vi "CARICA GRAFICI.vi"(0 "TRIFASE?":bool, 1 "N°curva":i32, 2 "TERMICA?":bool, 5 "indici":T2, 7 "CURVE SINGOLE IN":T3, 9 "dati":string[][](array[string]), 11 "filtra\nNPSH":bool, 12 "Cluster filtro":cluster{"index":i32, "length":i32}, 13 "Cluster":T1={"scelta grafico QH"=0, "scelta grafico QP"=1, "scelta grafico Qeta"=0, "scelta grafico temperature"=0} {"scelta grafico QH" items=["Q-Htot", "Q(n)-Htot(n)"]; "scelta grafico QP" items=["Q-P1", "Q-P2", "Q-P3", "Q(n)-P1(n)", "Q(n)-P2(n)", "Q(n)-P2(n Ps)", "Q(n)-P3(n)"]; "scelta grafico Qeta" items=["Q-EtaP", "Q-EtaGr", "Q(n)-Etap(n)", "Q(n)-EtaGr(n)"]; "scelta grafico temperature" items=["DT", "DTaux", "TC1", "TC2"]}, 14 "Grafico generico":cluster{"X":i32, "Y":i32}) -> (3 "Temperature":cluster{"X":dbl[], "Y":dbl[]}[](array[cluster]), 4 "Cluster graph":T4, 6 "curve idrauliche":cluster{"X":dbl[], "Y":dbl[]}[](array[cluster]), 8 "Collaudo da graficare":T3, 10 "rendimenti/Pot":cluster{"X":dbl[], "Y":dbl[]}[](array[cluster]), 15 "CURVE SINGOLE OUT":T3)   [LabVIEW 2019]
uses:
  TypeDef/Curve singole.ctl
  TypeDef/Indici.ctl
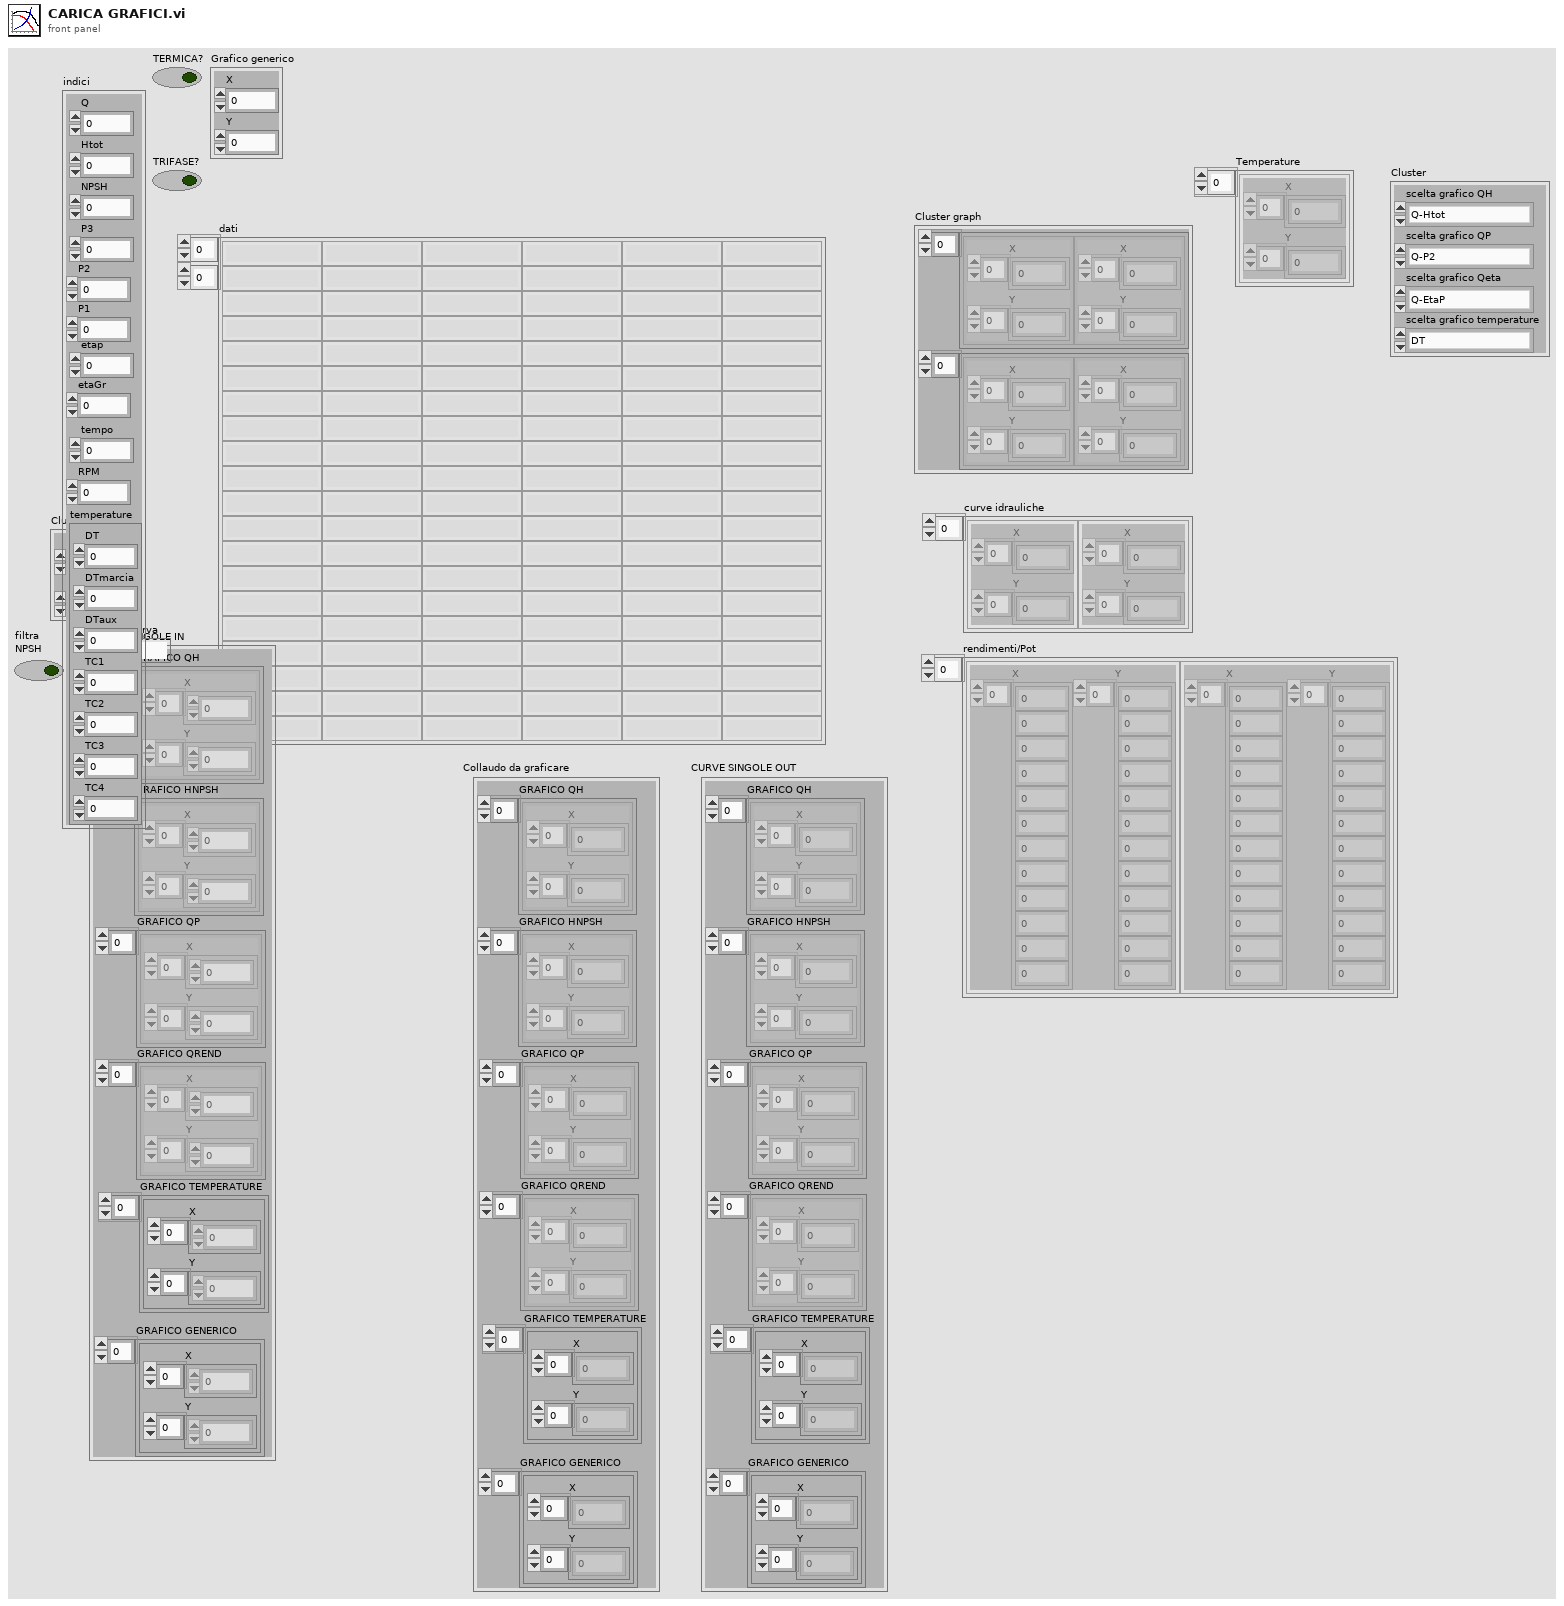
[diagram p1: front panel]
types:
  T1 = cluster{"scelta grafico QH":u16, "scelta grafico QP":u16, "scelta grafico Qeta":u16, "scelta grafico temperature":u16}
  T2 = typedef "Indici.ctl" = cluster{"Q":i32, "Htot":i32, "NPSH":i32, "P3":i32, "etap":i32, "temperature":cluster{"DT":i32, "DTmarcia":i32, "DTaux":i32, "TC1":i32, "TC2":i32, "TC3":i32, "TC4":i32}, "tempo":i32, "P2":i32, "P1":i32, "etaGr":i32, "RPM":i32}
  T3 = typedef "Curve singole.ctl" = cluster{"GRAFICO QH":cluster{"X":dbl[], "Y":dbl[]}[], "GRAFICO HNPSH":cluster{"X":dbl[], "Y":dbl[]}[], "GRAFICO QP":cluster{"X":dbl[], "Y":dbl[]}[], "GRAFICO QREND":cluster{"X":dbl[], "Y":dbl[]}[], "GRAFICO TEMPERATURE":cluster{"X":dbl[], "Y":dbl[]}[], "GRAFICO GENERICO":cluster{"X":dbl[], "Y":dbl[]}[]}
  T4 = cluster{cluster{"X":dbl[], "Y":dbl[]}[], cluster{"X":dbl[], "Y":dbl[]}[]}
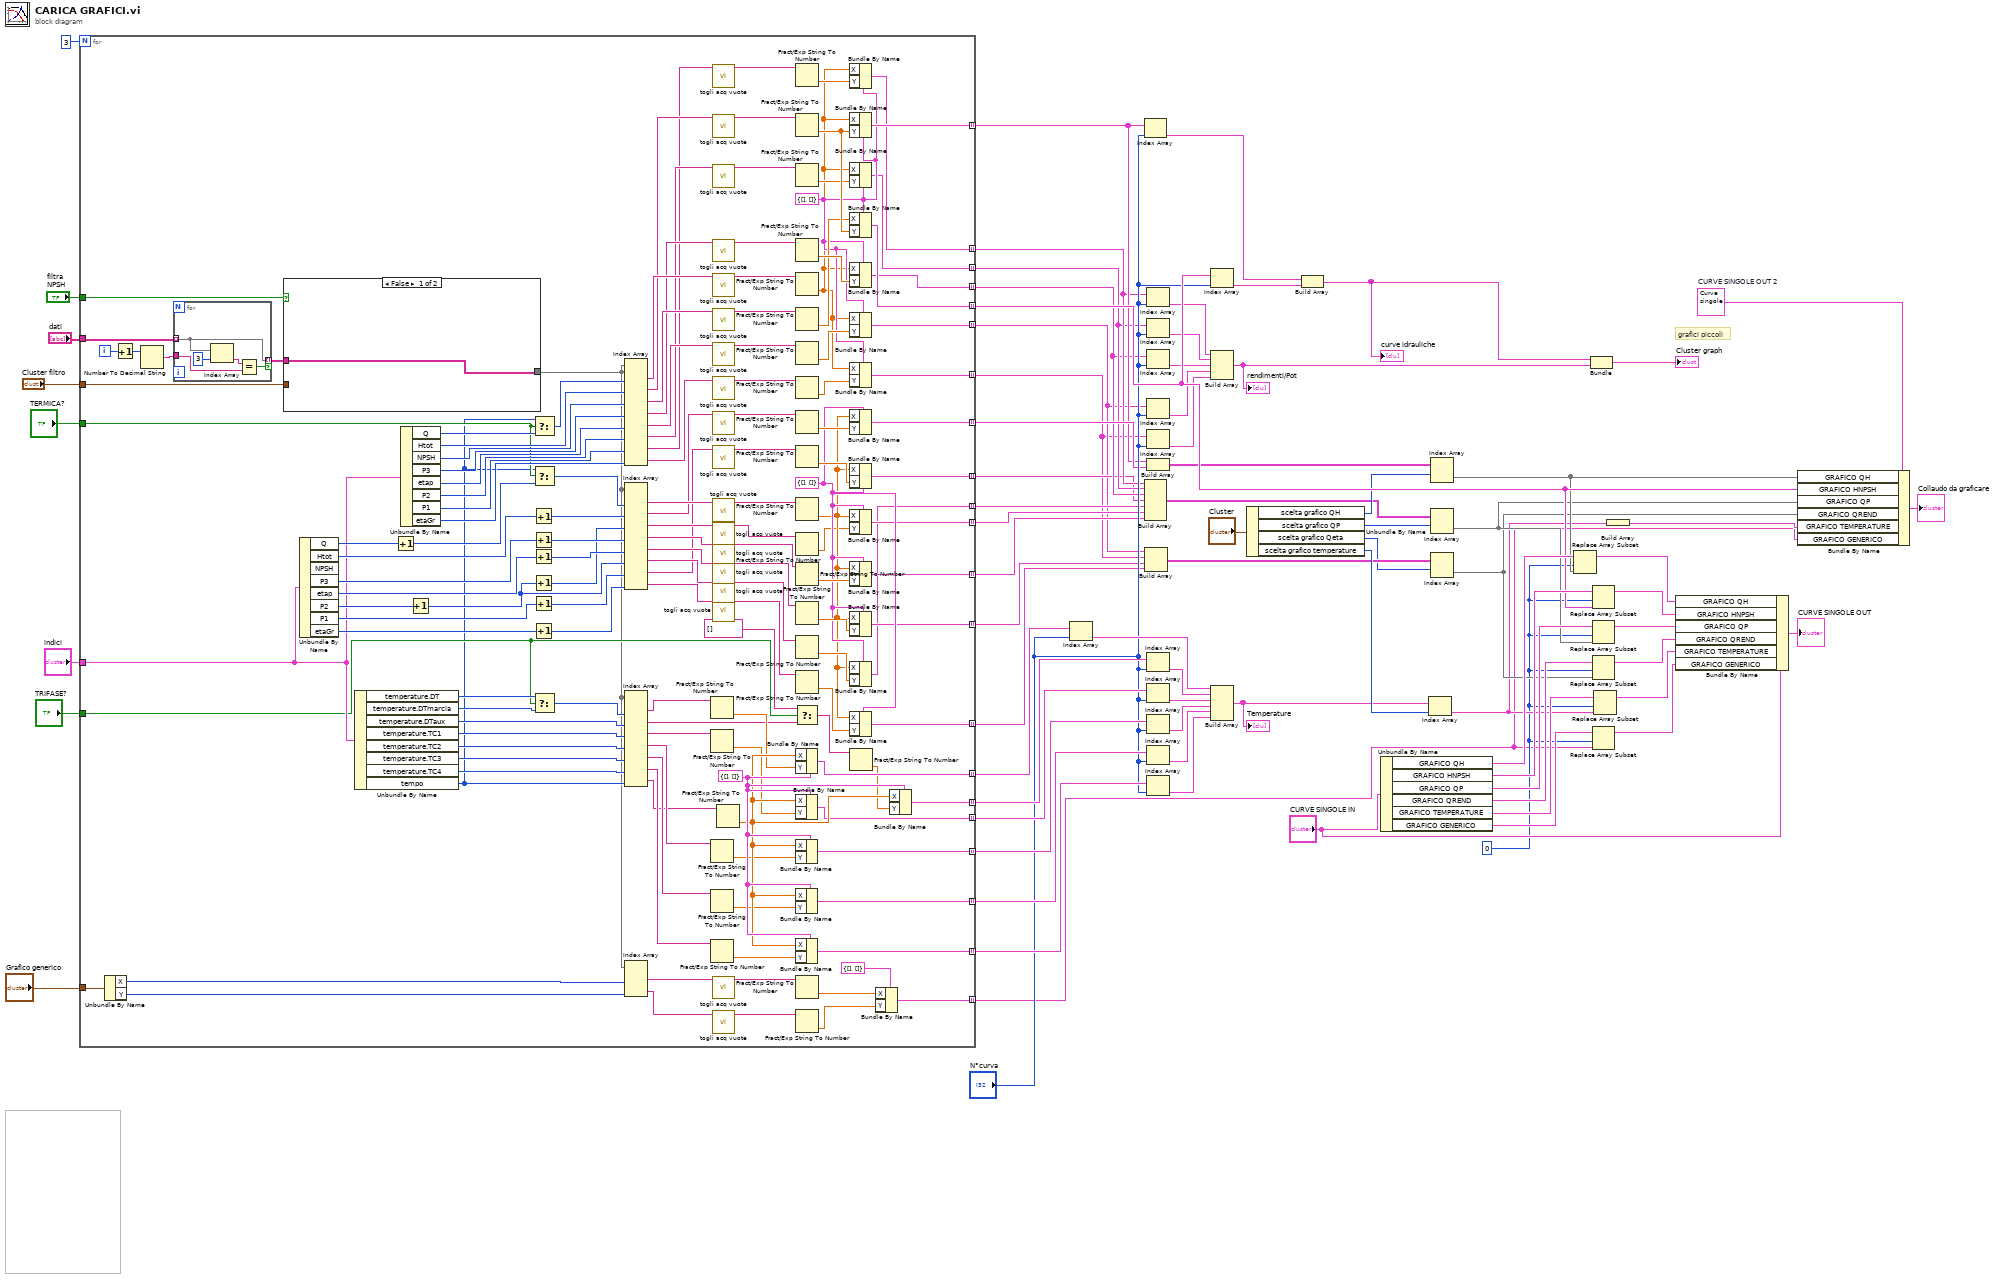
[diagram p0: block diagram]
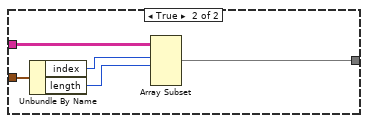
[diagram p2: hidden frame]
diagram:
  w62 = T3 {"GRAFICO QH"=[{"X"=[684.0, 638.0, 598.0, 565.0, 520.0, 479.0, 445.0, 405.0, 358.0, 320.0, 278.0, 238.0, 205.0, 157.0, 118.0, 81.0, 38.0, 0.0], "Y"=[7.0, 17.0, 24.0, 28.0, 34.0, 39.0, 42.0, 46.0, 50.0, 52.0, 54.0, 55.0, 56.0, 56.0, 56.0, 55.0, 54.0, 53.0]}], "GRAFICO HNPSH"=[{"X"=[], "Y"=[7.0, 17.0, 24.0, 28.0, 34.0, 39.0, 42.0, 46.0, 50.0, 52.0, 54.0, 55.0, 56.0, 56.0, 56.0, 55.0, 54.0, 53.0]}], "GRAFICO QP"=[{"X"=[684.0, 638.0, 598.0, 565.0, 520.0, 479.0, 445.0, 405.0, 358.0, 320.0, 278.0, 238.0, 205.0, 157.0, 118.0, 81.0, 38.0, 0.0], "Y"=[65816.0, 67180.0, 67438.0, 67220.0, 66491.0, 65328.0, 63977.0, 62006.0, 59186.0, 56284.0, 52488.0, 48222.0, 44877.0, 38995.0, 33621.0, 28828.0, 23844.0, 19872.0]}], "GRAFICO QREND"=[{"X"=[684.0, 638.0, 598.0, 565.0, 520.0, 479.0, 445.0, 405.0, 358.0, 320.0, 278.0, 238.0, 205.0, 157.0, 118.0, 81.0, 38.0, 0.0], "Y"=[20.0, 45.0, 58.0, 65.0, 73.0, 78.0, 80.0, 82.0, 82.0, 81.0, 78.0, 75.0, 70.0, 62.0, 53.0, 42.0, 23.0, 0.0]}], "GRAFICO TEMPERATURE"=[{"X"=[], "Y"=[]}, {"X"=[], "Y"=[]}, {"X"=[], "Y"=[]}, {"X"=[], "Y"=[]}, {"X"=[], "Y"=[]}, {"X"=[], "Y"=[]}, {"X"=[], "Y"=[]}, {"X"=[], "Y"=[]}, {"X"=[], "Y"=[]}, {"X"=[], "Y"=[]}, {"X"=[], "Y"=[]}, {"X"=[], "Y"=[]}, {"X"=[], "Y"=[]}, {"X"=[], "Y"=[]}, {"X"=[], "Y"=[]}, {"X"=[], "Y"=[]}, {"X"=[], "Y"=[]}, {"X"=[], "Y"=[]}, {"X"=[], "Y"=[]}, {"X"=[], "Y"=[]}, {"X"=[], "Y"=[]}, {"X"=[], "Y"=[]}, {"X"=[], "Y"=[]}, {"X"=[], "Y"=[]}, {"X"=[], "Y"=[]}, {"X"=[], "Y"=[]}, {"X"=[], "Y"=[]}, {"X"=[], "Y"=[]}, {"X"=[], "Y"=[]}, {"X"=[], "Y"=[]}, {"X"=[], "Y"=[]}, {"X"=[], "Y"=[]}, {"X"=[], "Y"=[]}, {"X"=[], "Y"=[]}, {"X"=[], "Y"=[]}, {"X"=[], "Y"=[]}, {"X"=[], "Y"=[]}, {"X"=[], "Y"=[]}, {"X"=[], "Y"=[]}, {"X"=[], "Y"=[]}, {"X"=[], "Y"=[]}, {"X"=[], "Y"=[]}, {"X"=[], "Y"=[]}, {"X"=[], "Y"=[]}, {"X"=[], "Y"=[]}, {"X"=[], "Y"=[]}, {"X"=[], "Y"=[]}, {"X"=[], "Y"=[]}, {"X"=[], "Y"=[]}, {"X"=[], "Y"=[]}], "GRAFICO GENERICO"=[{"X"=[], "Y"=[]}, {"X"=[], "Y"=[]}, {"X"=[], "Y"=[]}, {"X"=[], "Y"=[]}, {"X"=[], "Y"=[]}, {"X"=[], "Y"=[]}, {"X"=[], "Y"=[]}, {"X"=[], "Y"=[]}, {"X"=[], "Y"=[]}, {"X"=[], "Y"=[]}, {"X"=[], "Y"=[]}, {"X"=[], "Y"=[]}, {"X"=[], "Y"=[]}, {"X"=[], "Y"=[]}, {"X"=[], "Y"=[]}, {"X"=[], "Y"=[]}, {"X"=[], "Y"=[]}, {"X"=[], "Y"=[]}, {"X"=[], "Y"=[]}, {"X"=[], "Y"=[]}, {"X"=[], "Y"=[]}, {"X"=[], "Y"=[]}, {"X"=[], "Y"=[]}, {"X"=[], "Y"=[]}, {"X"=[], "Y"=[]}, {"X"=[], "Y"=[]}, {"X"=[], "Y"=[]}, {"X"=[], "Y"=[]}, {"X"=[], "Y"=[]}, {"X"=[], "Y"=[]}, {"X"=[], "Y"=[]}, {"X"=[], "Y"=[]}, {"X"=[], "Y"=[]}, {"X"=[], "Y"=[]}, {"X"=[], "Y"=[]}, {"X"=[], "Y"=[]}, {"X"=[], "Y"=[]}, {"X"=[], "Y"=[]}, {"X"=[], "Y"=[]}, {"X"=[], "Y"=[]}, {"X"=[], "Y"=[]}, {"X"=[], "Y"=[]}, {"X"=[], "Y"=[]}, {"X"=[], "Y"=[]}, {"X"=[], "Y"=[]}, {"X"=[], "Y"=[]}, {"X"=[], "Y"=[]}, {"X"=[], "Y"=[]}, {"X"=[], "Y"=[]}, {"X"=[], "Y"=[]}]}  # CURVE SINGOLE OUT 2
  w4 = 0 ("index")
  # "grafici piccoli"
  n1 = for {
    N: 3 -> [_]
    tunnel: "Cluster filtro" -> [w216]
    tunnel: "filtra\nNPSH" -> [w215]
    tunnel: [w214] -> w31 mode=indexing
    tunnel: [w213] -> w59 mode=indexing
    tunnel: [w212] -> w26 mode=indexing
    tunnel: [w211] -> w18 mode=indexing
    tunnel: "dati" -> [w210]
    tunnel: "indici" -> [w149]
    tunnel: [w188] -> w54 mode=indexing
    tunnel: [w187] -> w53 mode=indexing
    tunnel: [w186] -> w52 mode=indexing
    tunnel: [w185] -> w51 mode=indexing
    tunnel: [w184] -> w50 mode=indexing
    tunnel: [w183] -> w49 mode=indexing
    tunnel: [w165] -> w27 mode=indexing
    tunnel: [w164] -> w28 mode=indexing
    tunnel: [w163] -> w17 mode=indexing
    tunnel: [w138] -> w32 mode=indexing
    tunnel: [w137] -> w23 mode=indexing
    tunnel: [w136] -> w22 mode=indexing
    tunnel: [w135] -> w16 mode=indexing
    tunnel: [w134] -> w24 mode=indexing
    tunnel: [w133] -> w25 mode=indexing
    tunnel: [w132] -> w15 mode=indexing
    tunnel: "TRIFASE?" -> [w99]
    tunnel: "TERMICA?" -> [w94]
    tunnel: "Grafico generico" -> [w84]
    tunnel: [w81] -> w2 mode=indexing
    i -> [w209]
    w141 = cluster{"X":dbl[], "Y":dbl[]} {"X"=[], "Y"=[]}
    w190 = cluster{"X":dbl[], "Y":dbl[]} {"X"=[], "Y"=[]}
    w170 = cluster{"X":dbl[], "Y":dbl[]} {"X"=[], "Y"=[]}
    n2 = Unbundle By Name(w84) -> ("X"=w83:i32, "Y"=w82:i32)
    n3 = Increment(x=w209) -> (x+1=w80:i32)
    n4 = Number To Decimal String(number=w80) -> (decimal integer string=w79:string)  [unwired: 1 in]
    n5 = for {
      tunnel: w210 -> [w224] mode=indexing
      tunnel: w79 -> [w222]
      tunnel: [w224] -> w78 mode=indexing if=w225
      n6 = Index Array(array=w224, index=3) -> (element=w223:string)
      n7 = Equal?(x=w223, y=w222) -> (x = y?=w225:bool)
    }
    n8 = case shown="False" w215 {
      tunnel: w216 -> [_ w231]
      tunnel: w78 -> [w226 w230]
      tunnel: [w226 w227] -> w85
      frame False {
      }
      frame True {
        n9 = Unbundle By Name(w231) -> ("index"=w229:i32, "length"=w228:i32)
        n10 = Array Subset(array=w230, index (row)=w229, length (row)=w228) -> (w227:string[][])  [unwired: 2 in]
      }
    }
    n11 = Unbundle By Name(w149) -> ("Q"=w153:i32, "Htot"=w154:i32, "P3"=w155:i32, "etap"=w156:i32, "P2"=w157:i32, "P1"=w158:i32, "etaGr"=w159:i32)  [unwired: 1 out]
    n12 = Unbundle By Name(w149) -> ("temperature.DT"=w204:i32, "temperature.DTmarcia"=w203:i32, "temperature.DTaux"=w201:i32, "temperature.TC1"=w200:i32, "temperature.TC2"=w199:i32, "temperature.TC3"=w198:i32, "temperature.TC4"=w197:i32, "tempo"=w93:i32)
    n13 = Increment(x=w153) -> (x+1=w96:i32)
    n14 = Unbundle By Name(w149) -> ("Q"=w98:i32, "Htot"=w208:i32, "NPSH"=w207:i32, "P3"=w206:i32, "etap"=w205:i32, "P2"=w173:i32, "P1"=w172:i32, "etaGr"=w171:i32)
    n15 = Increment(x=w157) -> (x+1=w143:i32)
    n16 = Increment(x=w154) -> (x+1=w148:i32)
    n17 = Increment(x=w155) -> (x+1=w147:i32)
    n18 = Increment(x=w156) -> (x+1=w146:i32)
    n19 = Increment(x=w143) -> (x+1=w142:i32)
    n20 = Increment(x=w158) -> (x+1=w145:i32)
    n21 = Increment(x=w159) -> (x+1=w144:i32)
    n22 = Select(t=w93, s=w94, f=w98) -> (s? t:f=w97:i32)
    n23 = Select(t=w93, s=w94, f=w96) -> (s? t:f=w95:i32)
    n24 = Select(t=w204, s=w99, f=w203) -> (s? t:f=w202:i32)
    n25 = Index Array(array=w85, index (col) #1=w97, index (col) #2=w208, index (col) #3=w207, index (col) #4=w206, index (col) #5=w205, index (col) #6=w173, index (col) #7=w172, index (col) #8=w171) -> (element #1=w131:string[], element #2=w129:string[], element #3=w127:string[], element #4=w125:string[], element #5=w123:string[], element #6=w121:string[], element #7=w119:string[], element #8=w117:string[])  [unwired: 8 in]
    n26 = Index Array(array=w85, index (col) #1=w95, index (col) #2=w148, index (col) #3=w142, index (col) #4=w147, index (col) #5=w146, index (col) #6=w143, index (col) #7=w145, index (col) #8=w144) -> (element #1=w115:string[], element #2=w113:string[], element #3=w111:string[], element #4=w109:string[], element #5=w107:string[], element #6=w105:string[], element #7=w103:string[], element #8=w101:string[])  [unwired: 8 in]
    n27 = Index Array(array=w85, index (col) #1=w202, index (col) #2=w201, index (col) #3=w200, index (col) #4=w199, index (col) #5=w198, index (col) #6=w197, index (col) #7=w93) -> (element #1=w196:string[], element #2=w176:string[], element #3=w195:string[], element #4=w194:string[], element #5=w193:string[], element #6=w192:string[], element #7=w191:string[])  [unwired: 7 in]
    n28 = Index Array(array=w85, index (col) #1=w83, index (col) #2=w82) -> (element #1=w90:string[], element #2=w86:string[])  [unwired: 2 in]
    n29 = Fract/Exp String To Number(string=w196) -> (number=w182:dbl[])  [unwired: 3 in, 1 out]
    n30 = Fract/Exp String To Number(string=w195) -> (number=w180:dbl[])  [unwired: 3 in, 1 out]
    n31 = Fract/Exp String To Number(string=w194) -> (number=w179:dbl[])  [unwired: 3 in, 1 out]
    n32 = Fract/Exp String To Number(string=w193) -> (number=w178:dbl[])  [unwired: 3 in, 1 out]
    n33 = Fract/Exp String To Number(string=w192) -> (number=w177:dbl[])  [unwired: 3 in, 1 out]
    n34 = call "togli acq vuote.vi"("Q"=w119) -> ("Array"=w118:string[])  [unwired: 10 in]
    n35 = call "togli acq vuote.vi"("Q"=w129) -> ("Array"=w128:string[])  [unwired: 10 in]
    n36 = call "togli acq vuote.vi"("Q"=w121) -> ("Array"=w120:string[])  [unwired: 10 in]
    n37 = call "togli acq vuote.vi"("Q"=w125) -> ("Array"=w124:string[])  [unwired: 10 in]
    n38 = call "togli acq vuote.vi"("Q"=w131) -> ("Array"=w130:string[])  [unwired: 10 in]
    n39 = call "togli acq vuote.vi"("Q"=w127) -> ("Array"=w126:string[])  [unwired: 10 in]
    n40 = call "togli acq vuote.vi"("Q"=w123) -> ("Array"=w122:string[])  [unwired: 10 in]
    n41 = call "togli acq vuote.vi"("Q"=w117) -> ("Array"=w116:string[])  [unwired: 10 in]
    n42 = call "togli acq vuote.vi"("Q"=w113) -> ("Array"=w112:string[])  [unwired: 10 in]
    n43 = call "togli acq vuote.vi"("Q"=w103) -> ("Array"=w102:string[])  [unwired: 10 in]
    n44 = call "togli acq vuote.vi"("Q"=w115) -> ("Array"=w114:string[])  [unwired: 10 in]
    n45 = call "togli acq vuote.vi"("Q"=w111) -> ("Array"=w110:string[])  [unwired: 10 in]
    n46 = call "togli acq vuote.vi"("Q"=w109) -> ("Array"=w108:string[])  [unwired: 10 in]
    n47 = call "togli acq vuote.vi"("Q"=w107) -> ("Array"=w106:string[])  [unwired: 10 in]
    n48 = call "togli acq vuote.vi"("Q"=w105) -> ("Array"=w104:string[])  [unwired: 10 in]
    n49 = call "togli acq vuote.vi"("Q"=w101) -> ("Array"=w100:string[])  [unwired: 10 in]
    n50 = call "togli acq vuote.vi"("Q"=w90) -> ("Array"=w91:string[])  [unwired: 10 in]
    n51 = call "togli acq vuote.vi"("Q"=w86) -> ("Array"=w92:string[])  [unwired: 10 in]
    n52 = Fract/Exp String To Number(string=w191) -> (number=w189:dbl[])  [unwired: 3 in, 1 out]
    n53 = Fract/Exp String To Number(string=w118) -> (number=w168:dbl[])  [unwired: 3 in, 1 out]
    n54 = Fract/Exp String To Number(string=w128) -> (number=w218:dbl[])  [unwired: 3 in, 1 out]
    n55 = Fract/Exp String To Number(string=w120) -> (number=w169:dbl[])  [unwired: 3 in, 1 out]
    n56 = Fract/Exp String To Number(string=w124) -> (number=w219:dbl[])  [unwired: 3 in, 1 out]
    n57 = Fract/Exp String To Number(string=w130) -> (number=w166:dbl[])  [unwired: 3 in, 1 out]
    n58 = Fract/Exp String To Number(string=w126) -> (number=w217:dbl[])  [unwired: 3 in, 1 out]
    n59 = Fract/Exp String To Number(string=w122) -> (number=w220:dbl[])  [unwired: 3 in, 1 out]
    n60 = Fract/Exp String To Number(string=w116) -> (number=w167:dbl[])  [unwired: 3 in, 1 out]
    n61 = Fract/Exp String To Number(string=w112) -> (number=w152:dbl[])  [unwired: 3 in, 1 out]
    n62 = Fract/Exp String To Number(string=w102) -> (number=w161:dbl[])  [unwired: 3 in, 1 out]
    n63 = Fract/Exp String To Number(string=w114) -> (number=w140:dbl[])  [unwired: 3 in, 1 out]
    n64 = Fract/Exp String To Number(string=w110) -> (number=w139:dbl[])  [unwired: 3 in, 1 out]
    n65 = Fract/Exp String To Number(string=w108) -> (number=w151:dbl[])  [unwired: 3 in, 1 out]
    n66 = Fract/Exp String To Number(string=w106) -> (number=w150:dbl[])  [unwired: 3 in, 1 out]
    n67 = Fract/Exp String To Number(string=w104) -> (number=w160:dbl[])  [unwired: 3 in, 1 out]
    n68 = Fract/Exp String To Number(string=w100) -> (number=w162:dbl[])  [unwired: 3 in, 1 out]
    n69 = Select(t=string[] [], s=w99, f=w176) -> (s? t:f=w175:string[])
    n70 = Bundle By Name(cluster=w190, "X"=w189, "Y"=w182) -> (w188:cluster{"X":dbl[], "Y":dbl[]})
    n71 = Bundle By Name(cluster=w190, "X"=w189, "Y"=w180) -> (w186:cluster{"X":dbl[], "Y":dbl[]})
    n72 = Bundle By Name(cluster=w190, "X"=w189, "Y"=w179) -> (w185:cluster{"X":dbl[], "Y":dbl[]})
    n73 = Bundle By Name(cluster=w190, "X"=w189, "Y"=w178) -> (w184:cluster{"X":dbl[], "Y":dbl[]})
    n74 = Bundle By Name(cluster=w190, "X"=w189, "Y"=w177) -> (w183:cluster{"X":dbl[], "Y":dbl[]})
    n75 = Fract/Exp String To Number(string=w91) -> (number=w89:dbl[])  [unwired: 3 in, 1 out]
    n76 = Fract/Exp String To Number(string=w92) -> (number=w87:dbl[])  [unwired: 3 in, 1 out]
    n77 = Bundle By Name(cluster=w170, "X"=w166, "Y"=w168) -> (w164:cluster{"X":dbl[], "Y":dbl[]})
    n78 = Bundle By Name(cluster=w170, "X"=w166, "Y"=w218) -> (w214:cluster{"X":dbl[], "Y":dbl[]})
    n79 = Bundle By Name(cluster=w170, "X"=w166, "Y"=w169) -> (w165:cluster{"X":dbl[], "Y":dbl[]})
    n80 = Bundle By Name(cluster=w170, "X"=w217, "Y"=w218) -> (w213:cluster{"X":dbl[], "Y":dbl[]})
    n81 = Bundle By Name(cluster=w170, "X"=w166, "Y"=w219) -> (w212:cluster{"X":dbl[], "Y":dbl[]})
    n82 = Bundle By Name(cluster=w170, "X"=w166, "Y"=w220) -> (w211:cluster{"X":dbl[], "Y":dbl[]})
    n83 = Bundle By Name(cluster=w170, "X"=w166, "Y"=w167) -> (w163:cluster{"X":dbl[], "Y":dbl[]})
    n84 = Bundle By Name(cluster=w141, "X"=w140, "Y"=w152) -> (w138:cluster{"X":dbl[], "Y":dbl[]})
    n85 = Bundle By Name(cluster=w141, "X"=w140, "Y"=w161) -> (w133:cluster{"X":dbl[], "Y":dbl[]})
    n86 = Bundle By Name(cluster=w141, "X"=w140, "Y"=w139) -> (w137:cluster{"X":dbl[], "Y":dbl[]})
    n87 = Bundle By Name(cluster=w141, "X"=w140, "Y"=w151) -> (w136:cluster{"X":dbl[], "Y":dbl[]})
    n88 = Bundle By Name(cluster=w141, "X"=w140, "Y"=w150) -> (w135:cluster{"X":dbl[], "Y":dbl[]})
    n89 = Bundle By Name(cluster=w141, "X"=w140, "Y"=w160) -> (w134:cluster{"X":dbl[], "Y":dbl[]})
    n90 = Bundle By Name(cluster=w141, "X"=w140, "Y"=w162) -> (w132:cluster{"X":dbl[], "Y":dbl[]})
    n91 = Fract/Exp String To Number(string=w175) -> (number=w181:dbl[])  [unwired: 3 in, 1 out]
    n92 = Bundle By Name(cluster=cluster{"X":dbl[], "Y":dbl[]} {"X"=[], "Y"=[]}, "X"=w89, "Y"=w87) -> (w81:cluster{"X":dbl[], "Y":dbl[]})
    n93 = Bundle By Name(cluster=w190, "X"=w189, "Y"=w181) -> (w187:cluster{"X":dbl[], "Y":dbl[]})
  }
  n94 = Index Array(array=w54, index="N°curva") -> (element=w55:cluster{"X":dbl[], "Y":dbl[]})
  n95 = Index Array(array=w31, index="N°curva") -> (element=w33:cluster{"X":dbl[], "Y":dbl[]})
  n96 = Build Array(w28, w27, w26, w25, w24, w23, w22) -> (w21:cluster{"X":dbl[], "Y":dbl[]}[][])
  n97 = Build Array(w18, w17, w16, w15) -> (w14:cluster{"X":dbl[], "Y":dbl[]}[][])
  n98 = Index Array(array=w28, index="N°curva") -> (element=w44:cluster{"X":dbl[], "Y":dbl[]})
  n99 = Index Array(array=w27, index="N°curva") -> (element=w43:cluster{"X":dbl[], "Y":dbl[]})
  n100 = Index Array(array=w26, index="N°curva") -> (element=w45:cluster{"X":dbl[], "Y":dbl[]})
  n101 = Index Array(array=w18, index="N°curva") -> (element=w42:cluster{"X":dbl[], "Y":dbl[]})
  n102 = Index Array(array=w17, index="N°curva") -> (element=w41:cluster{"X":dbl[], "Y":dbl[]})
  n103 = Build Array(w31, w32) -> (w36:cluster{"X":dbl[], "Y":dbl[]}[][])
  n104 = Index Array(array=w53, index="N°curva") -> (element=w56:cluster{"X":dbl[], "Y":dbl[]})
  n105 = Index Array(array=w52, index="N°curva") -> (element=w48:cluster{"X":dbl[], "Y":dbl[]})
  n106 = Index Array(array=w51, index="N°curva") -> (element=w47:cluster{"X":dbl[], "Y":dbl[]})
  n107 = Index Array(array=w50, index="N°curva") -> (element=w46:cluster{"X":dbl[], "Y":dbl[]})
  n108 = Index Array(array=w49, index="N°curva") -> (element=w38:cluster{"X":dbl[], "Y":dbl[]})
  n109 = Index Array(array=w59, index="N°curva") -> (element=w60:cluster{"X":dbl[], "Y":dbl[]})
  n110 = Build Array(w44, w43, w45, w42, w41) -> (w76:cluster{"X":dbl[], "Y":dbl[]}[])
  "rendimenti/Pot" <- w76
  n111 = Build Array(w55, w56, w48, w47, w46, w38) -> (w34:cluster{"X":dbl[], "Y":dbl[]}[])
  "Temperature" <- w34
  n112 = Unbundle By Name("Cluster") -> ("scelta grafico QH"=w30:u16, "scelta grafico QP"=w20:u16, "scelta grafico Qeta"=w13:u16, "scelta grafico temperature"=w39:u16)
  n113 = Build Array(w33, w60) -> (w75:cluster{"X":dbl[], "Y":dbl[]}[])
  "curve idrauliche" <- w75
  n114 = Unbundle By Name("CURVE SINGOLE IN") -> ("GRAFICO QH"=w67:cluster{"X":dbl[], "Y":dbl[]}[], "GRAFICO HNPSH"=w68:cluster{"X":dbl[], "Y":dbl[]}[], "GRAFICO QP"=w69:cluster{"X":dbl[], "Y":dbl[]}[], "GRAFICO QREND"=w65:cluster{"X":dbl[], "Y":dbl[]}[], "GRAFICO TEMPERATURE"=w9:cluster{"X":dbl[], "Y":dbl[]}[], "GRAFICO GENERICO"=w6:cluster{"X":dbl[], "Y":dbl[]}[])
  n115 = Index Array(array=w34, index=w39) -> (element=w8:cluster{"X":dbl[], "Y":dbl[]})
  n116 = Index Array(array=w36, index (row)=w30) -> (element=w29:cluster{"X":dbl[], "Y":dbl[]}[])  [unwired: 1 in]
  n117 = Index Array(array=w21, index (row)=w20) -> (element=w19:cluster{"X":dbl[], "Y":dbl[]}[])  [unwired: 1 in]
  n118 = Index Array(array=w14, index (row)=w13) -> (element=w12:cluster{"X":dbl[], "Y":dbl[]}[])  [unwired: 1 in]
  n119 = Replace Array Subset "Replace Array Subset"(array=w67, new element=w29, index=w4) -> (w70:cluster{"X":dbl[], "Y":dbl[]}[])
  n120 = Bundle(w75, w76) -> (→"Cluster graph":T4)  [unwired: 1 in]
  n121 = Replace Array Subset(array=w68, new element=w59, index=w4) -> (w64:cluster{"X":dbl[], "Y":dbl[]}[])
  n122 = Replace Array Subset(array=w69, new element=w19, index=w4) -> (w71:cluster{"X":dbl[], "Y":dbl[]}[])
  n123 = Replace Array Subset(array=w65, new element=w12, index=w4) -> (w72:cluster{"X":dbl[], "Y":dbl[]}[])
  n124 = Replace Array Subset(array=w6, new element=w2, index=w4) -> (w5:cluster{"X":dbl[], "Y":dbl[]}[])
  n125 = Replace Array Subset(array=w9, new element=w8, index=w4) -> (w7:cluster{"X":dbl[], "Y":dbl[]}[])
  n126 = Build Array(w8) -> (w37:cluster{"X":dbl[], "Y":dbl[]}[])
  n127 = Bundle By Name(cluster="CURVE SINGOLE IN", "GRAFICO QH"=w70, "GRAFICO HNPSH"=w64, "GRAFICO QP"=w71, "GRAFICO QREND"=w72, "GRAFICO TEMPERATURE"=w7, "GRAFICO GENERICO"=w5) -> (→"CURVE SINGOLE OUT":T3)
  n128 = Bundle By Name(cluster=w62, "GRAFICO QH"=w29, "GRAFICO HNPSH"=w59, "GRAFICO QP"=w19, "GRAFICO QREND"=w12, "GRAFICO TEMPERATURE"=w37, "GRAFICO GENERICO"=w2) -> (→"Collaudo da graficare":T3)
